vi "_Test Process Debug Message Contains Message Handler Clone ID.vi"(8 "error in (no error)":errorcluster, 11 "Process Test In":refnum<class "Process Dev Test.lvclass">) -> (0 "error out":errorcluster, 3 "Process Test Out":refnum<class "Process Dev Test.lvclass">)   [LabVIEW 2020, in "Process Dev Test.lvclass"]
uses:
  Process Dev Test.lvclass
  C:/Program Files (x86)/National Instruments/LabVIEW 2020/vi.lib/Astemes/LUnit/Test Case.lvclass
  source/Framework Test Suite/Mock Process/Mock Process.lvclass
  C:/Git/astemes-triarc-framework/source/Framework/Process/Process.lvclass
  source/Framework/Process/Process.lvclass/Process.ctl
  <vilib>/Astemes/LUnit/Test Case.lvclass/Test Case.ctl
  <vilib>/Astemes/LUnit/LUnit Assertion Result.lvclass/LUnit Assertion Result.ctl
  <vilib>/Astemes/LUnit/LUnit Test Case Result.lvclass/LUnit Test Case Result.ctl
  <vilib>/Astemes/LUnit/LUnit Method Result.lvclass/LUnit Method Result.ctl
  source/Framework/Process/Private/SubVIs/Wait for finish.vi
  source/Framework/Process/Protected/Messaging/Enqueue Message.vi
  source/Framework/Process/Private/SubVIs/Set Lifecycle State.vi
  source/Framework/Process/Public/Lifecycle/Get Lifecycle State.vi
  <vilib>/Astemes/LUnit/Palette/Fail.vi
  <vilib>/Astemes/LUnit/Palette/Pass.vi
  <vilib>/Astemes/LUnit/Set Assertion Type.vi
  source/Framework/Process/Private/SubVIs/Handle Debug Data.vi
  <vilib>/Utility/error.llb/Clear Errors.vi
  <vilib>/Astemes/LUnit/Add test result.vi
  <vilib>/Astemes/LUnit/LUnit Write Passed.vi
  <vilib>/Astemes/LUnit/LUnit Write Message.vi
  <vilib>/Astemes/LUnit/LUnit Write Description.vi
  <vilib>/Astemes/LUnit/LUnit Write Assertion Type.vi
  source/Framework/Logging/Log Debug.vi
  <vilib>/AdvancedString/1D String Array to Delimited String.vi
  <vilib>/Utility/High Resolution Relative Seconds.vi
  <vilib>/Astemes/LUnit/LUnit Record Assertion Result.vi
  <vilib>/Astemes/LUnit/LUnit Aggregate Assertion Results.vi
  <vilib>/Astemes/LUnit/Assertion Result/LUnit Read Status.vi
  <vilib>/Astemes/LUnit/LUnit Read Message.vi
  <vilib>/Astemes/LUnit/LUnit Read Description.vi
  <vilib>/Astemes/LUnit/Method Result/LUnit Merge Status.vi
  <vilib>/Astemes/LUnit/LUnit Concatenate result strings.vi
  <vilib>/Utility/error.llb/Error Cluster From Error Code.vi
  source/Framework/Process/Public/Read Name.vi
  <vilib>/Astemes/LUnit/LUnit Assertion Result.lvclass
  source/Framework/Process/Process.lvclass
  Process Dev Test.lvclass/Process Dev Test.ctl
  <vilib>/Astemes/LUnit/Test Case.lvclass
panel:
  out "Call Chain":string
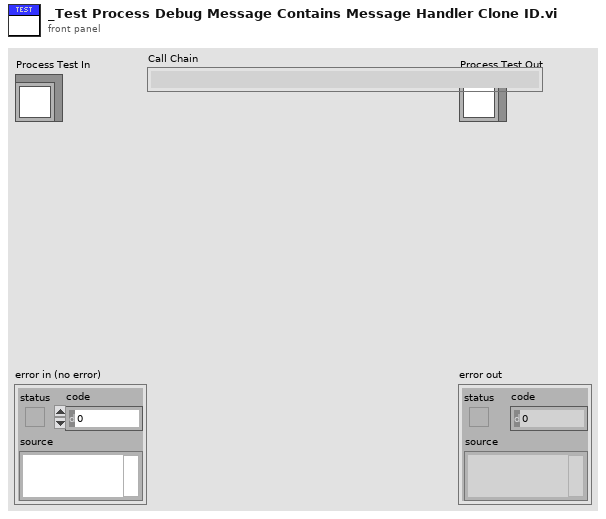
[diagram p1: front panel]
types:
  T1 = cluster{"Action":string, "Call Chain":string, "Process":string, "Message":string, "Message Data":variant, "Time":dbl}
  T2 = cluster{"Action":string, "Call Chain":string, "Process":string, "Message":string, "Message Data":variant, "Time":dbl}[]
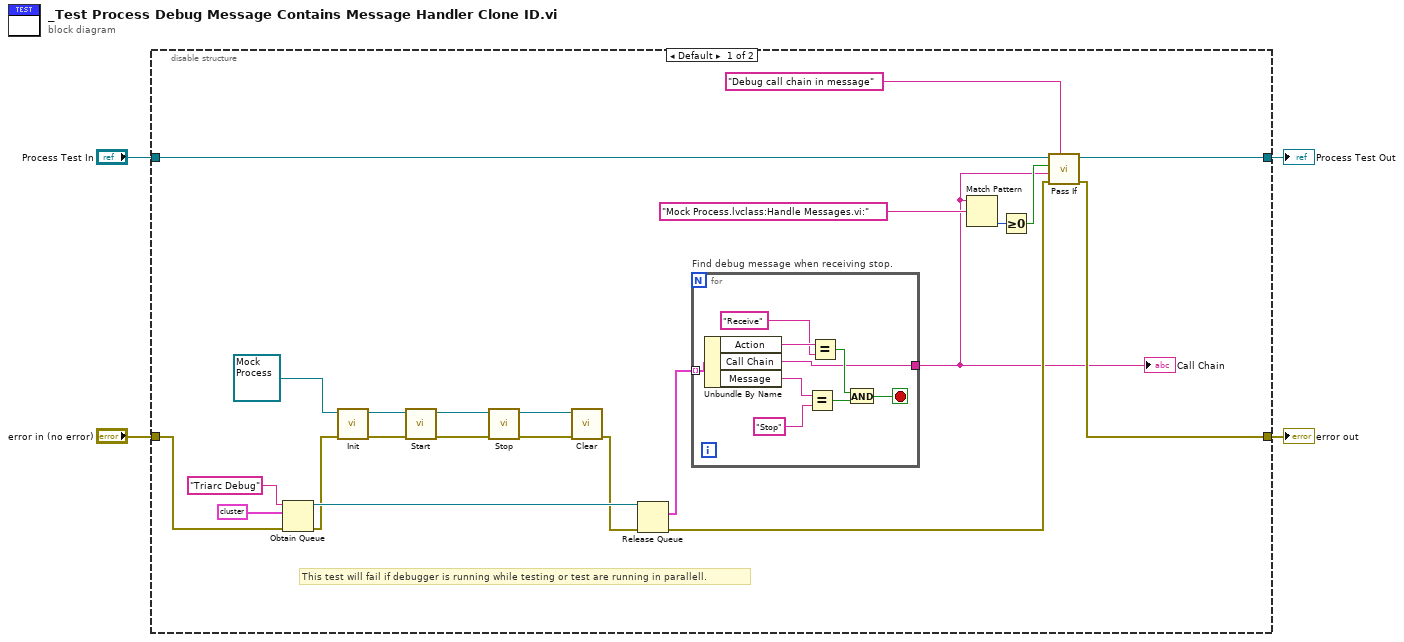
[diagram p0: block diagram]
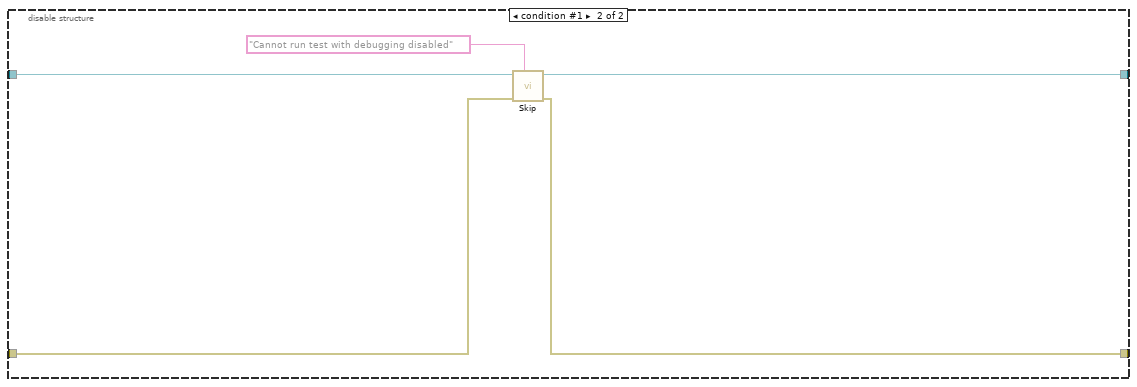
[diagram p2: hidden frame]
diagram:
  n1 = disable-structure shown="Default" {
    disable-tunnel: "Process Test In" -> [w27 w41]
    disable-tunnel: [w20 w39] -> w3
    disable-tunnel: [w19 w38] -> w2
    disable-tunnel: "error in (no error)" -> [w12 w40]
    frame condition #0 (active) {
      # "This test will fail if debugger is running while testing or test are running in parallell."
      n2 = Obtain Queue(name (unnamed)="Triarc Debug", element data type=T1 {"Action"="", "Call Chain"="", "Process"="", "Message"="", "Message Data"=variant, "Time"=0.0} ("output cluster"), error in (no error)=w12) -> (queue out=w15:refnum<queue>, error out=w13:errorcluster)  [unwired: 2 in, 1 out]
      n3 = call-dynamic "Init.vi"("error in (no error)"=w13, "Mock Process In"=refnum<class "Mock Process.lvclass"> refnum ("Mock Process.lvclass")) -> ("error out"=w26:errorcluster, "Mock Process Out"=w25:refnum<class "Mock Process.lvclass">)  [unwired: 8 in]
      n4 = call "Start.vi"("error in (no error)"=w26, "Process In"=w25) -> ("error out"=w23:errorcluster, "Process Out"=w24:refnum<class "Mock Process.lvclass">)  [unwired: 7 in, 1 out]
      n5 = call "Stop.vi"("error in (no error)"=w23, "Process In"=w24) -> ("error out"=w21:errorcluster, "Process Out"=w22:refnum<class "Mock Process.lvclass">)  [unwired: 7 in, 1 out]
      n6 = call-dynamic "Clear.vi"("error in (no error)"=w21, "Mock Process In"=w22) -> ("error out"=w11:errorcluster)  [unwired: 9 in]
      n7 = Release Queue(queue=w15, error in (no error)=w11) -> (remaining elements=w10:T2, error out=w9:errorcluster)  [unwired: 1 in, 1 out]
      n8 = for "Find debug message when receiving stop." {
        tunnel: w10 -> [w36] mode=indexing
        tunnel: [w28] -> w5
        stop <- w29 stop-if-true
        n9 = Unbundle By Name(w36) -> ("Action"=w32:string, "Call Chain"=w28:string, "Message"=w35:string)
        n10 = Equal?(x=w35, y="Stop") -> (x = y?=w33:bool)
        n11 = Equal?(x=w32, y="Receive") -> (x = y?=w30:bool)
        n12 = And(x=w30, y=w33) -> (x .and. y?=w29:bool)
      }
      "Call Chain" <- w5
      n13 = Match Pattern(string=w5, regular expression="Mock Process.lvclass:Handle Messages.vi:") -> (offset past match=w7:i32)  [unwired: 1 in, 3 out]
      n14 = Greater Or Equal To 0?(x=w7) -> (x >= 0?=w6:bool)
      n15 = call <vilib>:"Pass If.vi"("Description"="Debug call chain in message", "error in (no error)"=w9, "Message"=w5, "Pass?"=w6, "LUnit Test Case In"=w27) -> ("error out"=w19:errorcluster, "LUnit Test Case Out"=w20:refnum<class "Process Dev Test.lvclass">)  [unwired: 5 in]
    }
    frame condition #1 {
      n16 = call <vilib>:"Skip.vi"("Description"="Cannot run test with debugging disabled", "error in (no error)"=w40, "LUnit Test Case In"=w41) -> ("error out"=w38:errorcluster, "LUnit Test Case Out"=w39:refnum<class "Process Dev Test.lvclass">)  [unwired: 7 in]
    }
  }
  "error out" <- w2
  "Process Test Out" <- w3
